vi "simple Xcvr 2954 (Host).vi"() -> ()   [LabVIEW 2021]
uses:
  <vilib>/userdefined/High Color/nirio_resource_hc.ctl
  states.ctl
  <vilib>/Analysis/4window.llb/windowTd.ctl
  <vilib>/FPGAPlugInAG/USRP 294xR; 295xR 200 MSps/niLvFpga_Open_USRP 294xR; 295xR 200 MSps.vi
  <vilib>/rvi/interface/common/dynamic/niFpgaDynamicAddResources.vi
  <vilib>/Utility/error.llb/Error Cluster From Error Code.vi
  <vilib>/rvi/errors/niLvFpgaAdjustHostInterfaceError.vi
  <instrlib>/_niInstr/DSP/v1/FPGA/Public/Sub VIs/Data Conversion/U32 to IQ - 1 spc - S18.1.vi
  <vilib>/measure/maspectr.llb/FFT Spectrum (Mag-Phase) for 1 Chan (CDB).vi
  <vilib>/rvi/interface/nirviOpenFPGA/nirviOpenFPGA.xnode
  FPGA Bitfiles/simple  Xcvr (FPGA).lvbitx
  <vilib>/rvi/interface/nirviMethod/nirviMethod.xnode
  <vilib>/rvi/interface/nirviReadWriteControl/nirviReadWriteControl.xnode
  <instrlib>/niUsrpRio/Config/v1/Host/niUsrpRio Config v1 Host.lvlib
  <instrlib>/_niInstr/DSP/v1/FPGA/niInstr DSP v1 FPGA.lvlib
  <vilib>/Analysis/NI_AALPro.lvlib
  <vilib>/measure/NI_MAPro.lvlib
  <vilib>/rvi/interface/Simulation/niFpgaSimulationCallBeginRW.vi
  <vilib>/FPGAPlugInAG/Dynamic/niLvFpga_ReadFifo_Dynamic.vi
  <vilib>/rvi/errors/niLvFpgaMergeErrorWithErrorCode.vi
  NiFpgaLv.dll
  <vilib>/FPGAPlugInAG/Dynamic/niLvFpga_StartFifo_Dynamic.vi
panel:
  in  "DSP Rx params":T1(array[cluster])=[{"Frequency shift"=1000000.0, " sample rate"=5000000.0}, {"Frequency shift"=1000000.0, " sample rate"=10000000.0}] {"sample rate" min=-100000000.0 max=100000000.0 step=1000000.0 format="%#_6pHz"; "Frequency shift" min=-100000000.0 max=100000000.0 step=1000000.0 format="%#_6pHz"}
  out "scop":waveform(dbl)[](graph)=[{"t0"=timestamp(0 s since 1904-01-01), "dt"=2e-07, "Y"=array[8192 elements]}, {"t0"=timestamp(0 s since 1904-01-01), "dt"=1e-07, "Y"=array[8192 elements]}]
  out "spectrum":cluster{"f0":dbl, "df":dbl, "magnitude":dbl[]}[](graph)=[{"f0"=496500000.0, "df"=610.3515625, "magnitude"=array[8192 elements]}, {"f0"=494000000.0, "df"=1220.703125, "magnitude"=array[8192 elements]}]
  in  "resource name":T2="usrp"
  in  "DSP Tx params":cluster{"Tx Frequency":dbl, "Amplitude":dbl}[](array[cluster])=[{"Tx Frequency"=1000000.0, "Amplitude"=-20.0}, {"Tx Frequency"=1000000.0, "Amplitude"=-20.0}] {"Amplitude" min=-92.0 max=0.0 format="%#_6pdB"; "Tx Frequency" min=-100000000.0 max=100000000.0 step=1000000.0 format="%#_6pHz"}
  in  "RF Params":T3(array[cluster])=[{"Gain"=5.0, "frequency"=500000000.0, "enable ch 1"=TRUE}, {"Gain"=5.0, "frequency"=500000000.0, "enable ch 1"=TRUE}, {"Gain"=10.0, "frequency"=500000000.0, "enable ch 1"=TRUE}, {"Gain"=10.0, "frequency"=500000000.0, "enable ch 1"=TRUE}] {"frequency" min=10000000.0 max=6000000000.0 step=1000000.0 format="%#_6pHz"; "Gain" min=0.0 max=32.0 step=0.5 format="%#_6pdB"}
  in  "Max queue":i32=20
  in  "Number of Elements":u32=8192 step=1024
  out "Rx params":T4(array[cluster])=[{"Rx enable"=TRUE, "center frequncy"=496500000.0, "dt"=2e-07}, {"Rx enable"=TRUE, "center frequncy"=494000000.0, "dt"=1e-07}]
  # "USRP 2954 Tx / Rx HOST"
  # "Setup"
  # "Rx data"
  # "Device"
  # "Rx params"
  # "Tx params"
  # "CH0"
  # "CH1"
  # "CH0"
  # "CH1"
  # "RF params"
  # "DSP params"
  # "Computing"
  # "Channel 1 - 2 are not synced in this app"
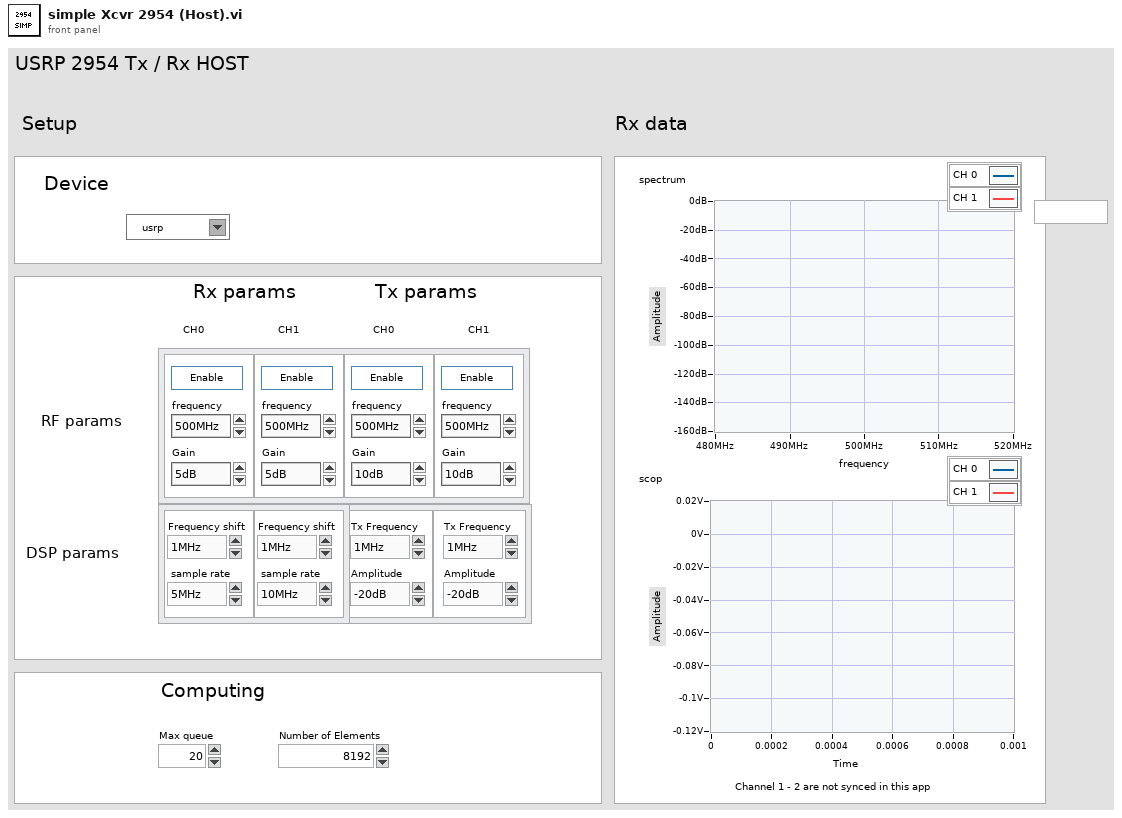
[diagram p1: front panel]
types:
  T1 = cluster{"Frequency shift":dbl, " sample rate":dbl}[]
  T2 = typedef "nirio_resource_hc.ctl" = tag
  T3 = cluster{"Gain":dbl, "frequency":dbl, "enable ch 1":bool}[]
  T4 = cluster{"Rx enable":bool, "center frequncy":dbl, "dt":dbl}[]
  T5 = typedef "states.ctl" = enum16{"ini", "set basic", "update DSP", "close sesion", "read", "wait"}
  T6 = enum16{"ini", "set basic", "update DSP", "close sesion"}
  T7 = cluster{"linear amp":fxp<+/-,18,1>, "frequency shift":fxp<+/-,48,0>}
  T8 = cluster{"Rx enable":bool, "center frequncy":dbl, "dt":dbl}
  T9 = cluster{"frequency shift":fxp<+/-,48,0>, "output sample rate":fxp<+,48,1>}
  T10 = typedef "niUsrpRio Config v1 Host.lvlib/niUsrpRio Session.ctl" = cluster{"FPGA Interface":refnum<k20>, "RIO Interface Number":u32, "Data Clock Rate":u32, "FPGA Data Clock Rate":u32, "Global Settings Register Bus":T11, "Radio 0 Settings Register Bus":T11, "Radio 1 Settings Register Bus":T11, "Radio Settings Bus Semaphore":T12, "DB Queues":T13[], "Characterization Data Valid?":bool, "EEPROM Header":T14, "Device Data Header":T15, "EEPROM Characterization Header":T16, "Characterization Data":T17[], "FPGA Current Version":u32, "FPGA Oldest Compatible Version":u32, "Fixed Logic Current Version":u32, "Fixed Logic Oldest Compatible Version":u32, "FPGA Radio Settings Bus Current Version":u32, "FPGA Radio Settings Bus Oldest Compatible Version":u32, "FPGA Board Config Current Version":u32, "FPGA Board Config Oldest Compatible Version":u32, "Daughterboard Clock Rate":u32, "daughterboard configuration session handles":u64[]}
  T11 = typedef "niInstr Register Bus v0 Host.lvlib/Register Bus Session.ctl" = refnum<queue>
  T12 = typedef "Semaphore RefNum" = refnum<k1>
  T13 = typedef "niUsrpRio Config v1 Host.lvlib/DB Queue Reference.ctl" = refnum<queue>
  T14 = typedef "niUsrpRio Config v1 Host.lvlib/EEPROM Header.ctl" = cluster{"Checksum":u32, "Product Code":u16, "Hardware Current Version":u16, "Hardware Oldest Compatible Version":u16, "EEPROM Map Current Version":u16, "EEPROM Map Oldest Compatible Version":u16, "User Password":string, "Pointer to Factory Header":u32, "Pointer to User Header":u32, "Recommended Interval":u16, "Number of Reserved Bytes":i32, "Number of Daughterboards":u8, "Daughterboard IDs":u16[], "Daughterboard Serial Numbers":string[]}
  T15 = typedef "niUsrpRio Config v1 Host.lvlib/EEPROM Device Data Header.ctl" = cluster{"Checksum":u32, "Number of Channels":u8, "Number of Gain Settings":u16[], "Pointer to Characterization Data":u32[], "Number of Reserved Bytes":i32, "Number of Frequencies":u16[]}
  T16 = typedef "niUsrpRio Config v1 Host.lvlib/EEPROM Characterization Header.ctl" = cluster{"Checksum":u32, "Date":timestamp, "Temperature":sgl, "Misc. Info":string, "Pointer to Device Data Header":u32, "Number of Reserved Bytes":i32}
  T17 = typedef "niUsrpRio Config v1 Host.lvlib/Characterization Data.ctl" = cluster{"Gains[dB]":dbl[], "Frequencies [Hz]":dbl[], "IQ Imbalance Table":T18[], "Measured Gains[dB]":dbl[][]}
  T18 = typedef "niUsrpRio Config v1 Host.lvlib/IQ Imbalance.ctl" = cluster{"Gain Imbalance [linear]":dbl, "Phase Imbalance [radians]":dbl, "Offset":cdb}
  T19 = typedef "niInstr DSP v1 Shared.lvlib/IQ Impairments.ctl" = cluster{"inline gain I":fxp<+/-,18,1>, "inline gain Q":fxp<+/-,18,1>, "cross gain I":fxp<+/-,18,1>, "cross gain Q":fxp<+/-,18,1>, "pre-gain offset I":fxp<+/-,18,1>, "pre-gain offset Q":fxp<+/-,18,1>, "post-gain offset I":fxp<+/-,18,1>, "post-gain offset Q":fxp<+/-,18,1>}
  T20 = cluster{"dB On (F)":bool, "unwrap phase (F)":bool, "convert to degree (F)":bool}
  T21 = typedef "NI_AALPro.lvlib/windowTd.ctl" = u32
  T22 = typedef "niInstr DSP v1 Shared.lvlib/IQ Data.ctl" = cluster{"I":fxp<+/-,18,1>, "Q":fxp<+/-,18,1>, "overflow":bool}
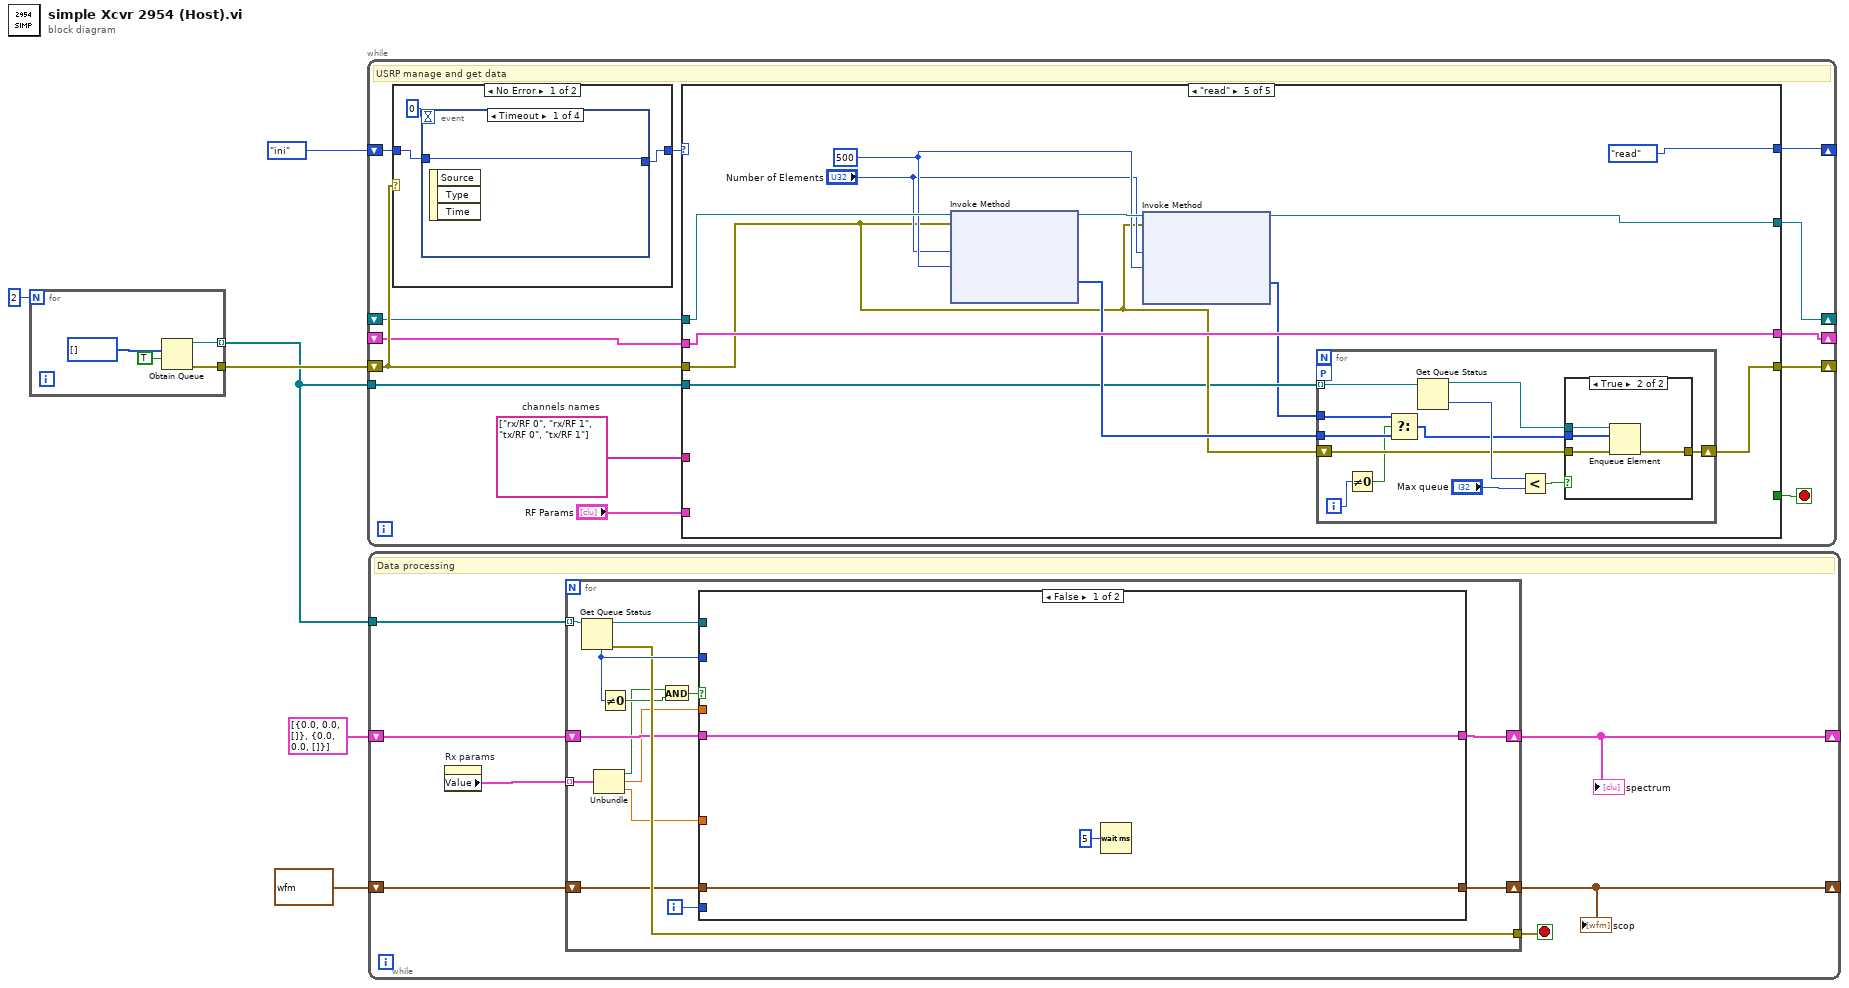
[diagram p0: block diagram]
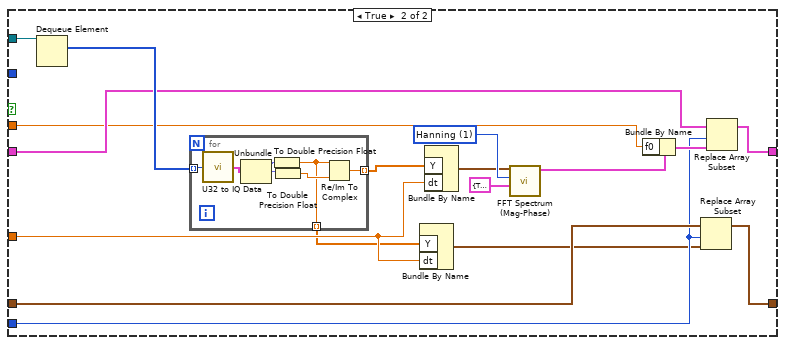
[diagram p2: hidden frame]
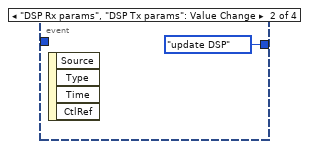
[diagram p3: hidden frame]
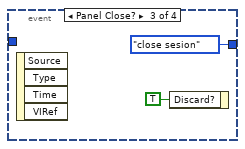
[diagram p4: hidden frame]
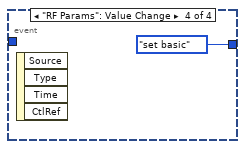
[diagram p5: hidden frame]
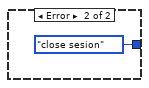
[diagram p6: hidden frame]
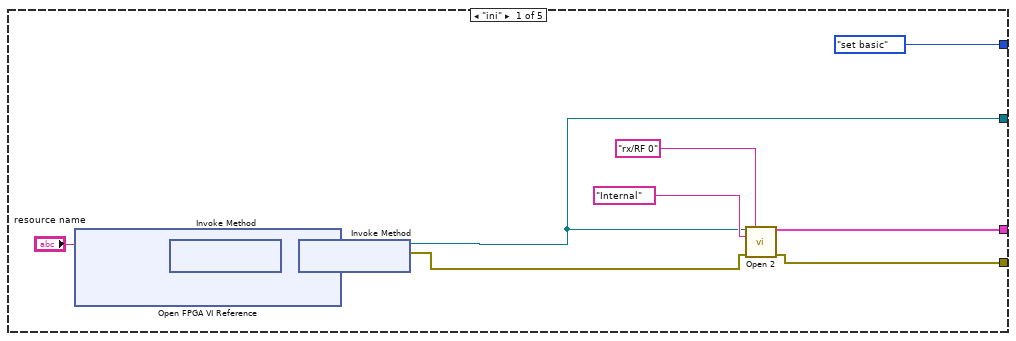
[diagram p7: hidden frame]
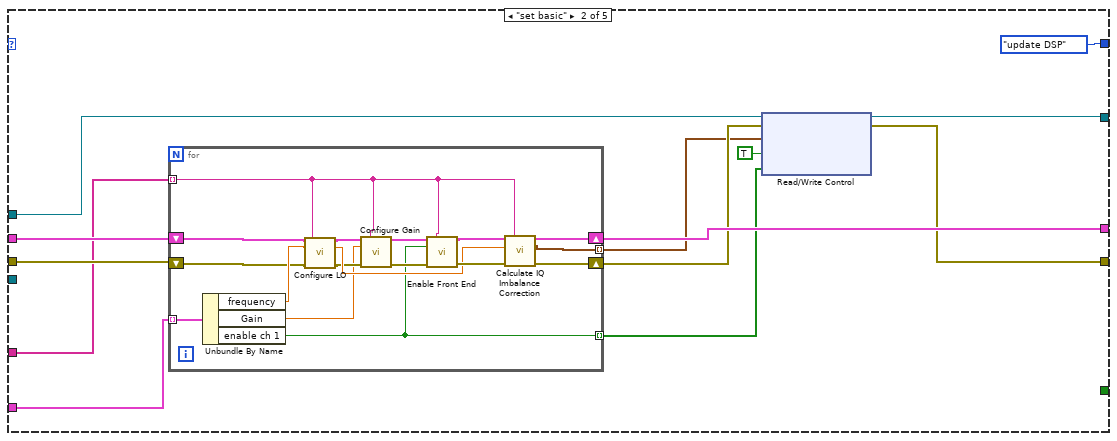
[diagram p8: hidden frame]
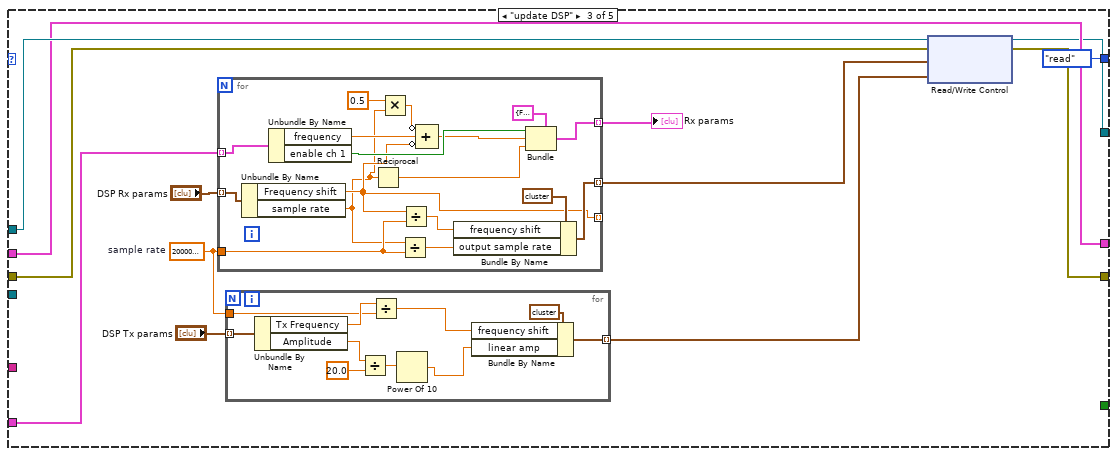
[diagram p9: hidden frame]
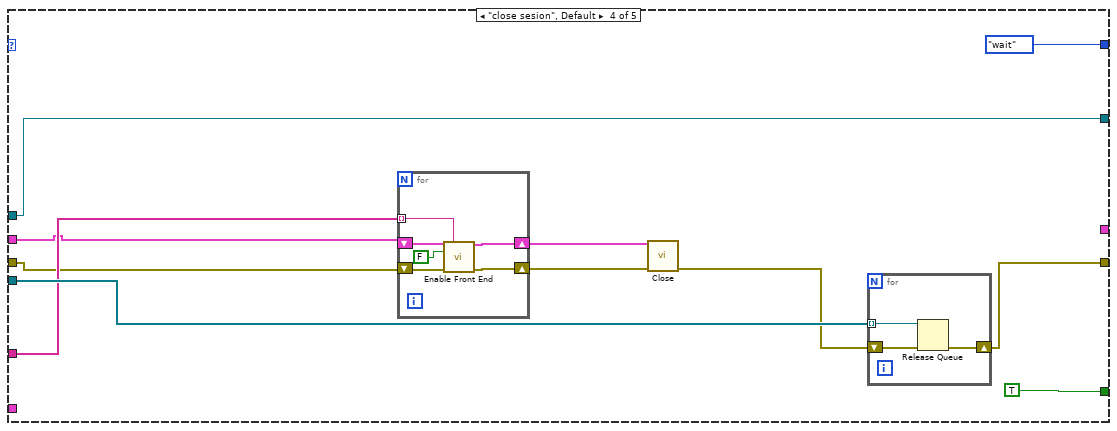
[diagram p10: hidden frame]
diagram:
  n1 = for {
    N: 2 -> [_]
    tunnel: [w9] -> w5
    tunnel: [w7] -> w4 mode=indexing
    n2 = Obtain Queue(element data type=u32[] [] ("Data"), create if not found? (T)=TRUE) -> (queue out=w7:refnum<queue>, error out=w9:errorcluster)  [unwired: 3 in, 1 out]
  }
  n3 = while {
    shift-right: [w16] -> _
    shift-left: states."ini" -> [w23]
    shift-right: [w13] -> _
    shift-left: _ -> [w17]
    shift-right: [w21] -> _
    shift-left: _ -> [w18]
    shift-right: [w20] -> _
    shift-left: w5 -> [w19]
    tunnel: w4 -> [w14]
    stop <- w15 stop-if-true
    w12 = string[] ["rx/RF 0", "rx/RF 1", "tx/RF 0", "tx/RF 1"]  # channels names
    # "USRP manage and get data"
    n4 = case shown="No Error" w19 {
      tunnel: w23 -> [w25 _]
      tunnel: [w24 T6."close sesion"] -> w22
      frame No Error {
        n5 = event shown="[0] Timeout" {
          selector: _ -> [_ _ _ _]
          dyn-events: _ -> [_ _ _ _]
          timeout: 0 -> [_ _ _ _]
          tunnel: w25 -> [w27 _ _ _]
          tunnel: [w27 states."update DSP" states."close sesion" states."set basic"] -> w24
          event Timeout {
            n6 = event-data() -> ()  [unwired: 1 in, 3 out]
          }
          event "DSP Rx params", "DSP Tx params": Value Change {
            n7 = event-data() -> ()  [unwired: 1 in, 4 out]
          }
          event Panel Close? {
            n8 = event-data() -> ()  [unwired: 1 in, 4 out]
            n9 = event-data("Discard?"=TRUE) -> ()  [unwired: 1 in, 1 out]
          }
          event "RF Params": Value Change {
            n10 = event-data() -> ()  [unwired: 1 in, 4 out]
          }
        }
      }
      frame Error {
      }
    }
    n11 = case shown="\"read\"" w22 {
      tunnel: [w42 w55 w85 _ w146] -> w21
      tunnel: [w41 w51 w84 w121 w138] -> w20
      tunnel: w19 -> [_ w57 w86 w117 w137]
      tunnel: w18 -> [_ w56 w85 w118 w146]
      tunnel: w17 -> [_ w53 w87 w120 w144]
      tunnel: [states."set basic" states."update DSP" states."read" states."wait" states."read"] -> w16
      tunnel: [_ _ _ TRUE _] -> w15
      tunnel: w14 -> [_ _ _ w123 w136]
      tunnel: [w33 w50 w77 w120 w139] -> w13
      tunnel: w12 -> [_ w47 _ w119 _]
      tunnel: "RF Params" -> [_ w46 w76 _ _]
      frame "ini" {
        n12 = xnode "Open FPGA VI Reference"("resource name"="resource name") -> ("FPGA VI Reference Out"=w34:refnum<k20>, "error out"=w36:errorcluster)  [unwired: 1 in]
        n13 = xnode "Invoke Method"("FPGA VI Reference In"=w34, "error in"=w36) -> ("FPGA VI Reference Out"=w38:refnum<k20>, "error out"=w37:errorcluster)
        n14 = xnode "Invoke Method"("FPGA VI Reference In"=w38, "error in"=w37) -> ("FPGA VI Reference Out"=w33:refnum<k20>, "error out"=w35:errorcluster)
        n15 = call <instrlib>:"Open 2.vi"("fpga ref"=w33, "scope"="rx/RF 0", "Reference Frequency Source"="Internal", "error in"=w35) -> ("niUsrpRio Session (out)"=w42:T10, "error out"=w41:errorcluster)  [unwired: 10 in]
      }
      frame "set basic" {
        n16 = for {
          shift-right: [w73] -> w55
          shift-left: w56 -> [w67]
          shift-right: [w72] -> w52
          shift-left: w57 -> [w65]
          tunnel: w47 -> [w62] mode=indexing
          tunnel: w46 -> [w74] mode=indexing
          tunnel: [w71] -> w49 mode=indexing
          tunnel: [w58] -> w45 mode=indexing
          n17 = Unbundle By Name(w74) -> ("frequency"=w66:dbl, "Gain"=w59:dbl, "enable ch 1"=w58:bool)
          n18 = call <instrlib>:"Configure LO.vi"("niUsrpRio Session"=w67, "scope"=w62, "frequency"=w66, "error in"=w65) -> ("niUsrpRio Session (out)"=w61:T10, "coerced frequency"=w68:dbl, "error out"=w60:errorcluster)  [unwired: 8 in, 1 out]
          n19 = call <instrlib>:"Configure Gain.vi"("niUsrpRio Session"=w61, "scope"=w62, "gain"=w59, "error in"=w60) -> ("niUsrpRio Session (out)"=w63:T10, "error out"=w64:errorcluster)  [unwired: 9 in, 1 out]
          n20 = call <instrlib>:"Enable Front End.vi"("niUsrpRio Session"=w63, "scope"=w62, "enable"=w58, "error in"=w64) -> ("niUsrpRio Session (out)"=w69:T10, "error out"=w70:errorcluster)  [unwired: 10 in]
          n21 = call <instrlib>:"Calculate IQ Imbalance Correction.vi"("niUsrpRio Session"=w69, "scope"=w62, "frequency"=w68, "error in"=w70) -> ("niUsrpRio Session (out)"=w73:T10, "IQ imbalance correction"=w71:T19, "error out"=w72:errorcluster)  [unwired: 8 in, 1 out]
        }
        n22 = xnode "Read/Write Control"("FPGA VI Reference In"=w53, "error in"=w52, "impairments"=w49, "start trigger"=TRUE, "send data to host"=w45) -> ("FPGA VI Reference Out"=w50:refnum<k20>, "error out"=w51:errorcluster)
      }
      frame "update DSP" {
        w80 = 200000000.0  # sample rate
        n23 = for {
          tunnel: "DSP Rx params" -> [w112] mode=indexing
          tunnel: [w114] -> w81 mode=indexing
          tunnel: w80 -> [w110]
          tunnel: [w101] -> _ mode=indexing
          tunnel: w76 -> [w108] mode=indexing
          tunnel: [w102] -> w75 mode=indexing
          n24 = Unbundle By Name(w112) -> ("Frequency shift"=w101:dbl, "sample rate"=w99:dbl)
          n25 = Unbundle By Name(w108) -> ("frequency"=w104:dbl, "enable ch 1"=w106:bool)
          n26 = Reciprocal(x=w99) -> (1/x=w105:dbl)
          n27 = Multiply(x=0.5, y=w99) -> (x*y=w98:dbl)
          n28 = Divide(x=w99, y=w110) -> (x/y=w113:dbl)
          n29 = Divide(x=w101, y=w110) -> (x/y=w109:dbl)
          n30 = Compound Arithmetic op=ADD(invert w98, w104, invert w101) -> (w103:dbl)
          n31 = Bundle By Name(cluster=T9 {"frequency shift"=0.0, "output sample rate"=0.0} ("DDC params"), "frequency shift"=w109, "output sample rate"=w113) -> (w114:T9)
          n32 = Bundle(cluster=T8 {"Rx enable"=FALSE, "center frequncy"=0.0, "dt"=0.0} ("Rx params"), "Rx enable"=w106, "center frequncy"=w103, "dt"=w105) -> (w102:T8)
        }
        "Rx params" <- w75
        n33 = for {
          tunnel: "DSP Tx params" -> [w96] mode=indexing
          tunnel: [w97] -> w78 mode=indexing
          tunnel: w80 -> [w93]
          n34 = Unbundle By Name(w96) -> ("Tx Frequency"=w95:dbl, "Amplitude"=w94:dbl)
          n35 = Divide(x=w94, y=20.0) -> (x/y=w90:dbl)
          n36 = Divide(x=w95, y=w93) -> (x/y=w92:dbl)
          n37 = Power Of 10(x=w90) -> (10^x=w88:dbl)
          n38 = Bundle By Name(cluster=T7 {"linear amp"=0.0, "frequency shift"=0.0} ("Tx params"), "frequency shift"=w92, "linear amp"=w88) -> (w97:T7)
        }
        n39 = xnode "Read/Write Control"("FPGA VI Reference In"=w87, "error in"=w86, "DDC params"=w81, "Tx params"=w78) -> ("FPGA VI Reference Out"=w77:refnum<k20>, "error out"=w84:errorcluster)
      }
      frame "close sesion", Default {
        n40 = for {
          tunnel: w119 -> [w131] mode=indexing
          shift-right: [w127] -> w116
          shift-left: w118 -> [w129]
          shift-right: [w126] -> w115
          shift-left: w117 -> [w128]
          n41 = call <instrlib>:"Enable Front End.vi"("niUsrpRio Session"=w129, "scope"=w131, "enable"=FALSE, "error in"=w128) -> ("niUsrpRio Session (out)"=w127:T10, "error out"=w126:errorcluster)  [unwired: 10 in]
        }
        n42 = call <instrlib>:"Close.vi"("niUsrpRio Session"=w116, "error in"=w115) -> ("error out"=w122:errorcluster)  [unwired: 12 in, 1 out]
        n43 = for {
          tunnel: w123 -> [w134] mode=indexing
          shift-right: [w132] -> w121
          shift-left: w122 -> [w133]
          n44 = Release Queue(queue=w134, error in (no error)=w133) -> (error out=w132:errorcluster)  [unwired: 1 in, 2 out]
        }
      }
      frame "read" {
        w141 = 500 ("Timeout (ms)")
        n45 = xnode "Invoke Method"("FPGA VI Reference In"=w144, "error in"=w137, "Number of Elements"="Number of Elements", "Timeout (ms)"=w141) -> ("FPGA VI Reference Out"=w142:refnum<k20>, "Data"=w143:u32[])  [unwired: 2 out]
        n46 = xnode "Invoke Method"("FPGA VI Reference In"=w142, "error in"=w137, "Number of Elements"="Number of Elements", "Timeout (ms)"=w141) -> ("FPGA VI Reference Out"=w139:refnum<k20>, "Data"=w135:u32[])  [unwired: 2 out]
        n47 = for {
          tunnel: w143 -> [w149]
          shift-right: [w154] -> w138
          shift-left: w137 -> [w153]
          tunnel: w136 -> [w152] mode=indexing
          tunnel: w135 -> [w150]
          workers-P: _ -> [_]
          i -> [w151]
          n48 = Not Equal To 0?(x=w151) -> (x != 0?=w147:bool)
          n49 = Select(t=w150, s=w147, f=w149) -> (s? t:f=w148:u32[])
          n50 = Get Queue Status(queue=w152) -> (queue out=w158:refnum<queue>, # elements in queue=w157:i32)  [unwired: 2 in, 6 out]
          n51 = Less?(x=w157, y="Max queue") -> (x < y?=w156:bool)
          n52 = case shown="True" w156 {
            tunnel: w148 -> [_ w160]
            tunnel: w153 -> [w159 w163]
            tunnel: [w159 w162] -> w154
            tunnel: w158 -> [_ w161]
            frame False {
              # "#add coment"
            }
            frame True {
              n53 = Enqueue Element(queue=w161, element=w160, error in (no error)=w163) -> (error out=w162:errorcluster)  [unwired: 1 in, 2 out]
            }
          }
        }
      }
    }
  }
  n54 = while {
    tunnel: w4 -> [w170]
    shift-right: [w167] -> _
    shift-left: cluster{"f0":dbl, "df":dbl, "magnitude":dbl[]}[] [{"f0"=0.0, "df"=0.0, "magnitude"=[]}, {"f0"=0.0, "df"=0.0, "magnitude"=[]}] -> [w166]
    shift-right: [w165] -> _
    shift-left: waveform(dbl)[] [{"t0"=timestamp(0 s since 1904-01-01), "dt"=1.0, "Y"=[]}, {"t0"=timestamp(0 s since 1904-01-01), "dt"=1.0, "Y"=[1.0]}] -> [w164]
    stop <- w169 stop-if-true
    # "Data processing"
    n55 = property on="Rx params" class="Arr (strict)"() -> ("Value"=w168:T4)  [unwired: 2 in, 2 out]
    n56 = for {
      tunnel: w170 -> [w183] mode=indexing
      tunnel: [w182] -> w169
      shift-right: [w178] -> w167
      shift-left: w166 -> [w179]
      shift-right: [w177] -> w165
      shift-left: w164 -> [w181]
      tunnel: w168 -> [w174] mode=indexing
      i -> [w180]
      n57 = Get Queue Status(queue=w183) -> (queue out=w185:refnum<queue>, error out=w182:errorcluster, # elements in queue=w184:i32)  [unwired: 2 in, 5 out]
      n58 = Unbundle(w174) -> ("Rx enable"=w173:bool, "center frequncy"=w172:dbl, "dt"=w171:dbl)
      n59 = Not Equal To 0?(x=w184) -> (x != 0?=w176:bool)
      n60 = And(x=w173, y=w176) -> (x .and. y?=w175:bool)
      n61 = case shown="False" w175 {
        tunnel: w184 -> [_ _]
        tunnel: w185 -> [_ w205]
        tunnel: w171 -> [_ w192]
        tunnel: w181 -> [w186 w200]
        tunnel: w180 -> [_ w196]
        tunnel: [w186 w199] -> w177
        tunnel: w179 -> [w187 w198]
        tunnel: [w187 w195] -> w178
        tunnel: w172 -> [_ w189]
        frame False {
          n62 = Wait (ms)(milliseconds to wait=u32 5) -> ()  [unwired: 1 out]
        }
        frame True {
          w203 = T21 1 items=["Rectangle"=0, "Hanning"=1, "Hamming"=2, "Blackman-Harris"=3, "Exact Blackman"=4, "Blackman"=5, "Flat Top"=6, "4 Term B-Harris "=7, "7 Term B-Harris"=8, "Low Sidelobe"=9, "Blackman Nuttall"=11, "Triangle"=30, "Bartlett-Hanning"=31, "Bohman"=32, "Parzen"=33, "Welch"=34, "Kaiser"=60, "Dolph-Chebyshev"=61, "Gaussian"=62] ("window")
          n63 = Dequeue Element(queue=w205) -> (element=w204:u32[])  [unwired: 2 in, 3 out]
          n64 = for {
            tunnel: w204 -> [w212] mode=indexing
            tunnel: [w210] -> w193 mode=indexing
            tunnel: [w206] -> w191 mode=indexing
            n65 = call-poly <instrlib>:"U32 to IQ Data.vi"("U32 data"=w212) -> ("IQ data"=w211:T22)  [unwired: 14 in]
            n66 = Unbundle(w211) -> ("I"=w209:fxp<+/-,18,1>, "Q"=w208:fxp<+/-,18,1>)  [unwired: 1 out]
            n67 = To Double Precision Float(number=w209) -> (double precision float=w206:dbl)
            n68 = To Double Precision Float(number=w208) -> (double precision float=w207:dbl)
            n69 = Re/Im To Complex(1:w207, 2:w206) -> (0:w210:cdb)
          }
          n70 = Bundle By Name("Y"=w191, "dt"=w192) -> (w190:waveform(dbl))  [unwired: 1 in]
          n71 = Bundle By Name("Y"=w193, "dt"=w192) -> (w194:waveform(cdb))  [unwired: 1 in]
          n72 = call-poly <vilib>:"FFT Spectrum (Mag-Phase).vi"("view"=T20 {"dB On (F)"=TRUE, "unwrap phase (F)"=FALSE, "convert to degree (F)"=TRUE}, "window"=w203, "time signal"=w194) -> ("magnitude"=w201:cluster{"f0":dbl, "df":dbl, "magnitude":dbl[]})  [unwired: 4 in, 4 out]
          n73 = Bundle By Name(cluster=w201, "f0"=w189) -> (w197:cluster{"f0":dbl, "df":dbl, "magnitude":dbl[]})
          n74 = Replace Array Subset(array=w200, new element=w190, index=w196) -> (w199:waveform(dbl)[])
          n75 = Replace Array Subset(array=w198, new element=w197, index=w196) -> (w195:cluster{"f0":dbl, "df":dbl, "magnitude":dbl[]}[])
        }
      }
    }
    "scop" <- w165
    "spectrum" <- w167
  }
